vi "Pulse Config Chan.vi"(8 "error in (no error)":errorcluster, 10 "Channel (1)":u32=1, 11 "3300 in":refnum<class "3300.lvclass">) -> (0 "error out":errorcluster, 3 "3300 out":refnum<class "3300.lvclass">)   [LabVIEW 2019, in "3300.lvlib" / "3300.lvclass"]
uses:
  Library/3300.lvclass
  Library/3300.lvclass/3300.ctl
  Accessors/Write Local Resource.vi
  <instrlib>/Agilent N330X Series/Agilent N330X Series.lvlib
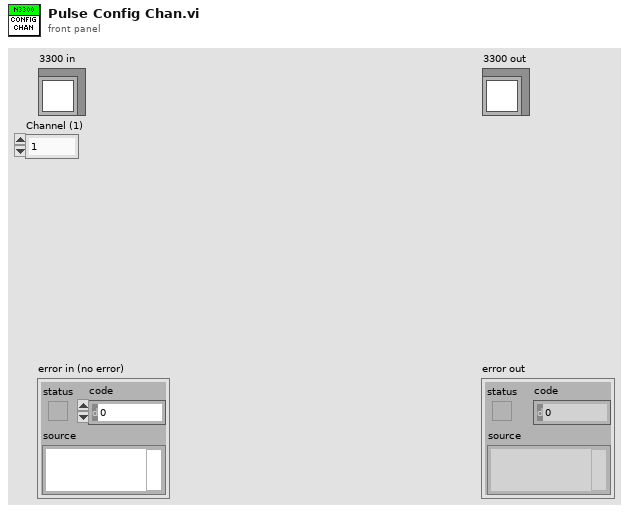
[diagram p1: front panel]
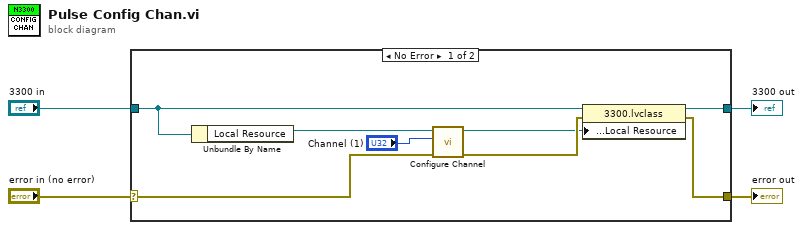
[diagram p0: block diagram]
diagram:
  n1 = case shown="No Error" "error in (no error)" {
    selector: "error in (no error)" -> [w5 w14]
    tunnel: [w8 w14] -> w3
    tunnel: [w7 w13] -> w1
    tunnel: "3300 in" -> [w11 w13]
    frame No Error {
      n2 = Unbundle By Name(w11) -> ("Local Resource"=w10:refnum<visa-resource-name>)
      n3 = call <instrlib>:"Configure Channel.vi"("error in (no error)"=w5, "Channel (1)"="Channel (1)", "VISA resource name"=w10) -> ("error out"=w9:errorcluster, "VISA resource name out"=w6:refnum<visa-resource-name>)  [unwired: 7 in]
      n4 = property class="3300.lvclass"(reference=w11, error in=w9, "Private:Accessors:Local Resource"=w6) -> (reference out=w7:refnum<class "3300.lvclass">, error out=w8:errorcluster)
    }
    frame Error {
    }
  }
  "error out" <- w3
  "3300 out" <- w1
